vi "Graph.vi"(8 "error in (no error)":errorcluster, 11 "Message Queues":T1) -> ()   [LabVIEW 2023, in "Weather Monitor Views.lvlib"]
doc: "Calls the Weather Monitor web service with different content-types and displays the raw data that is returned."
uses:
  Weather Monitor Views.lvlib
  support/Message Queue/All Message Queues.ctl
  support/Message Queue/Message Cluster.ctl
  Request/Response Data.ctl
  <vilib>/wsapi/NI_WebServices.lvlib
  support/Message Queue/Weather Message Queue.lvlib
  Weather Request Loop.lvlib
  support/User Event - Stop/Weather User Event - Stop.lvlib
panel:
  in  "Close button":bool
  out "Weather data":picture
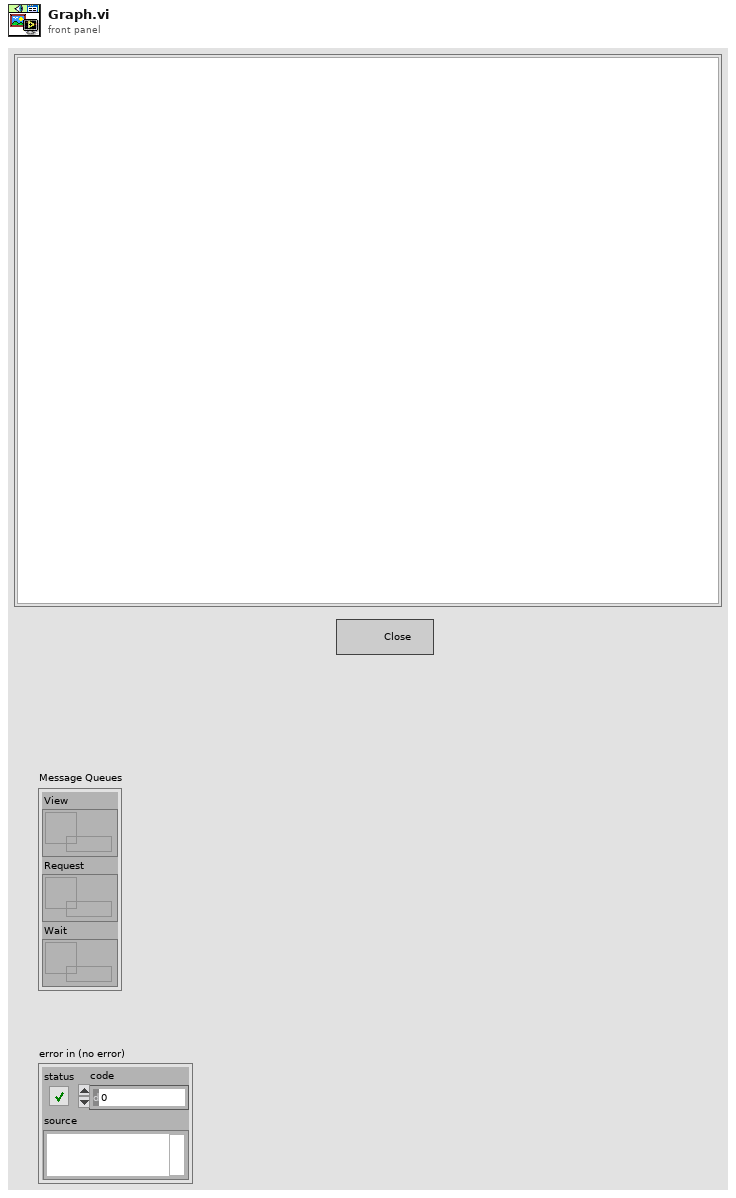
[diagram p1: front panel]
types:
  T1 = typedef "Weather Message Queue.lvlib/All Message Queues.ctl" = cluster{"View":refnum<queue>, "Request":refnum<queue>, "Wait":refnum<queue>}
  T2 = typedef "Weather Request Loop.lvlib/Response Data.ctl" = cluster{"Response Code":u16, "Body":string, "Headers":variant, "error":errorcluster}
  T3 = typedef "imagedata.ctl" = cluster{"image type":i32, "image depth":i32, "image":u8[], "mask":u8[], "colors":u32[], "Rectangle":cluster{"left":i16, "top":i16, "right":i16, "bottom":i16}}
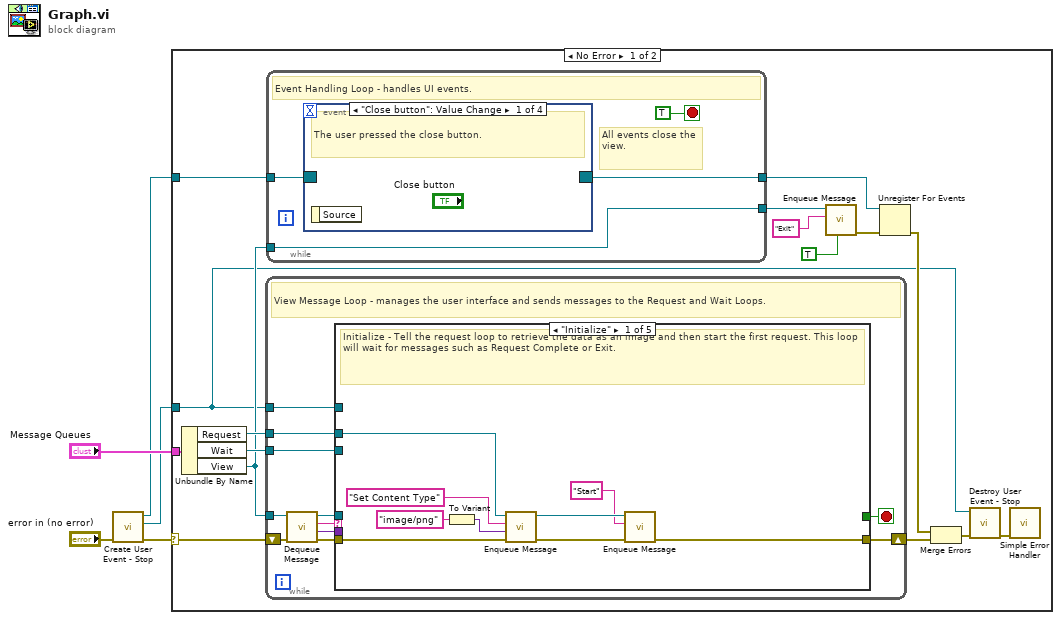
[diagram p0: block diagram]
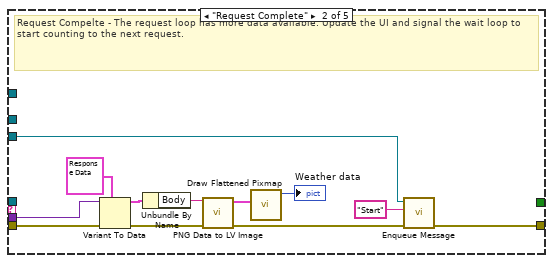
[diagram p2: hidden frame]
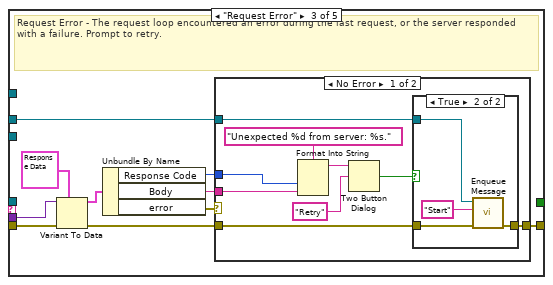
[diagram p3: hidden frame]
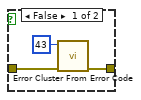
[diagram p4: hidden frame]
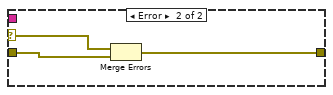
[diagram p5: hidden frame]
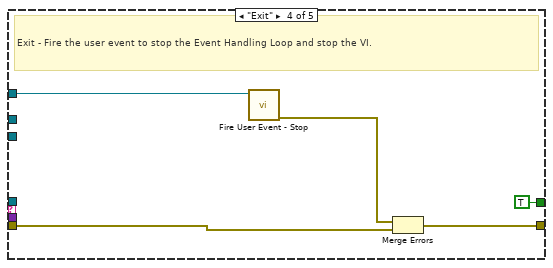
[diagram p6: hidden frame]
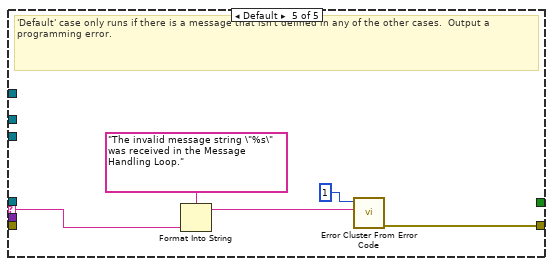
[diagram p7: hidden frame]
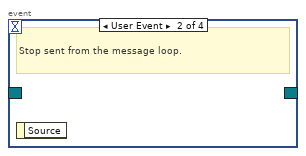
[diagram p8: hidden frame]
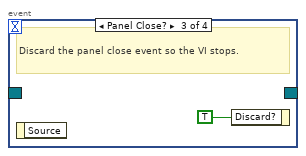
[diagram p9: hidden frame]
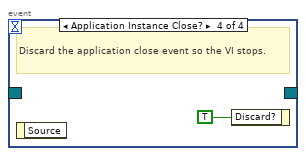
[diagram p10: hidden frame]
diagram:
  n1 = call "Create User Event - Stop.vi"("error in (no error)"="error in (no error)") -> ("error out"=w3:errorcluster, "User Event - Stop"=w1:refnum<user-event>, "Stop Event Registration Refnum"=w2:refnum<event-registration>)  [unwired: 8 in]
  n2 = case shown="No Error" w3 {
    selector: w3 -> [w16 _]
    tunnel: "Message Queues" -> [w21 _]
    tunnel: w2 -> [w15 _]
    tunnel: w1 -> [w10 _]
    frame No Error {
      n3 = Unbundle By Name(w21) -> ("Request"=w20:refnum<queue>, "Wait"=w19:refnum<queue>, "View"=w18:refnum<queue>)
      n4 = while {
        tunnel: w20 -> [w24]
        tunnel: w19 -> [w25]
        tunnel: w18 -> [w32]
        shift-right: [w26] -> w17
        shift-left: w16 -> [w31]
        tunnel: w10 -> [w22]
        stop <- w23 stop-if-true
        # "View Message Loop - manages the user interface and sends messages to the Request and Wait Loops."
        n5 = call "Dequeue Message.vi"("error in (no error)"=w31, "Message Queue"=w32) -> ("error out"=w27:errorcluster, "Message Data"=w28:variant, "Message"=w30:string, "dup Message Queue"=w29:refnum<queue>)  [unwired: 6 in]
        n6 = case shown="\"Initialize\"" w30 {
          selector: w30 -> [_ _ _ _ w89]
          tunnel: w29 -> [_ _ _ _ _]
          tunnel: w28 -> [_ w52 w62 _ _]
          tunnel: w27 -> [w41 w53 w63 w83 _]
          tunnel: [w33 w44 w55 w84 w88] -> w26
          tunnel: w25 -> [_ w43 _ _ _]
          tunnel: w24 -> [w40 _ w54 _ _]
          tunnel: [_ _ _ TRUE _] -> w23
          tunnel: w22 -> [_ _ _ w86 _]
          frame "Initialize" {
            # "Initialize - Tell the request loop to retrieve the data as an image and then start the first request. This loop will wait for messages such as Request Complete or Exit."
            n7 = To Variant(anything="image/png") -> (Variant=w37:variant)
            n8 = call "Enqueue Message.vi"("error in (no error)"=w41, "Message Data"=w37, "Message"="Set Content Type", "Message Queue"=w40) -> ("error out"=w35:errorcluster, "dup Message Queue"=w36:refnum<queue>)  [unwired: 6 in]
            n9 = call "Enqueue Message.vi"("error in (no error)"=w35, "Message"="Start", "Message Queue"=w36) -> ("error out"=w33:errorcluster)  [unwired: 7 in, 1 out]
          }
          frame "Request Complete" {
            # "Request Compelte - The request loop has more data available. Update the UI and signal the wait loop to start counting to the next request."
            n10 = Variant To Data(error in=w53, type=T2 {"Response Code"=0, "Body"="", "Headers"=variant, "error"={"status"=FALSE, "code"=0, "source"=""}} ("Response Data"), Variant=w52) -> (data=w48:T2, error out=w46:errorcluster)
            n11 = Unbundle By Name(w48) -> ("Body"=w47:string)
            n12 = call <vilib>:"PNG Data to LV Image.vi"("error in (no error)"=w46, "png data"=w47) -> ("error out"=w45:errorcluster, "image data"=w50:T3)  [unwired: 8 in]
            n13 = call <vilib>:"Draw Flattened Pixmap.vi"("image data"=w50) -> ("new picture"=→"Weather data":picture)  [unwired: 8 in]
            n14 = call "Enqueue Message.vi"("error in (no error)"=w45, "Message"="Start", "Message Queue"=w43) -> ("error out"=w44:errorcluster)  [unwired: 7 in, 1 out]
          }
          frame "Request Error" {
            # "Request Error - The request loop encountered an error during the last request, or the server responded with a failure. Prompt to retry."
            n15 = Variant To Data(error in=w63, type=T2 {"Response Code"=0, "Body"="", "Headers"=variant, "error"={"status"=FALSE, "code"=0, "source"=""}} ("Response Data"), Variant=w62) -> (data=w60:T2, error out=w57:errorcluster)
            n16 = Unbundle By Name(w60) -> ("Response Code"=w59:u16, "Body"=w58:string, "error"=w56:errorcluster)
            n17 = case shown="No Error" w56 {
              selector: w56 -> [_ w82]
              tunnel: w59 -> [w69 _]
              tunnel: w58 -> [w68 _]
              tunnel: w57 -> [w67 w80]
              tunnel: [w66 w81] -> w55
              tunnel: w54 -> [w65 _]
              frame No Error {
                n18 = Format Into String(format string="Unexpected %d from server: %s.", w69, w68) -> (resulting string=w71:string)  [unwired: 2 in, 1 out]
                n19 = Two Button Dialog(message=w71, 2:"Retry" ("T button name (\"OK\")")) -> (T button?=w64:bool)  [unwired: 1 in]
                n20 = case shown="True" w64 {
                  tunnel: w67 -> [w74 w79]
                  tunnel: [w75 w78] -> w66
                  tunnel: w65 -> [_ w77]
                  frame False {
                    n21 = call <vilib>:"Error Cluster From Error Code.vi"("error in (no error)"=w74, "error code (0)"=43) -> ("error out"=w75:errorcluster)  [unwired: 7 in]
                  }
                  frame True {
                    n22 = call "Enqueue Message.vi"("error in (no error)"=w79, "Message"="Start", "Message Queue"=w77) -> ("error out"=w78:errorcluster)  [unwired: 7 in, 1 out]
                  }
                }
              }
              frame Error {
                n23 = Merge Errors(w82, w80) -> (w81:errorcluster)
              }
            }
          }
          frame "Exit" {
            # "Exit - Fire the user event to stop the Event Handling Loop and stop the VI."
            n24 = call "Fire User Event - Stop.vi"("User Event - Stop"=w86) -> ("error out"=w85:errorcluster)  [unwired: 10 in]
            n25 = Merge Errors(w85, w83) -> (w84:errorcluster)
          }
          frame Default {
            # "'Default' case only runs if there is a message that isn't defined in any of the other cases.  Output a programming error."
            n26 = Format Into String(format string="The invalid message string \"%s\" was received in the Message Handling Loop." ("Unknown Message Error Text"), w89) -> (resulting string=w90:string)  [unwired: 2 in, 1 out]
            n27 = call <vilib>:"Error Cluster From Error Code.vi"("error message (\"\")"=w90, "error code (0)"=1) -> ("error out"=w88:errorcluster)  [unwired: 7 in]
          }
        }
      }
      n28 = while {
        tunnel: w18 -> [w93]
        tunnel: w15 -> [w95]
        tunnel: [w94] -> w13
        tunnel: [w93] -> w6
        stop <- TRUE stop-if-true
        # "All events close the view."
        # "Event Handling Loop - handles UI events."
        n29 = event shown="[0] \"Close button\": Value Change" {
          selector: w95 -> [_ _ _ _]
          dyn-events: [_ _ _ _] -> w94
          timeout: _ -> [_ _ _ _]
          event "Close button": Value Change {
            # "The user pressed the close button."
            n30 = event-data() -> ()  [unwired: 1 in, 1 out]
          }
          event User Event {
            # "Stop sent from the message loop."
            n31 = event-data() -> ()  [unwired: 1 in, 1 out]
          }
          event Panel Close? {
            # "Discard the panel close event so the VI stops."
            n32 = event-data() -> ()  [unwired: 1 in, 1 out]
            n33 = event-data("Discard?"=TRUE) -> ()  [unwired: 1 in, 1 out]
          }
          event Application Instance Close? {
            # "Discard the application close event so the VI stops."
            n34 = event-data() -> ()  [unwired: 1 in, 1 out]
            n35 = event-data("Discard?"=TRUE) -> ()  [unwired: 1 in, 1 out]
          }
        }
      }
      n36 = call "Enqueue Message.vi"("Priority Message? (F)"=TRUE, "Message"="Exit", "Message Queue"=w6) -> ("error out"=w7:errorcluster)  [unwired: 7 in, 1 out]
      n37 = Unregister For Events(event registration refnum=w13, error in=w7) -> (error out=w14:errorcluster)
      n38 = Merge Errors(w14, w17) -> (w12:errorcluster)
      n39 = call "Destroy User Event - Stop.vi"("error in (no error)"=w12, "User Event - Stop"=w10) -> ("error out"=w11:errorcluster)  [unwired: 9 in]
      n40 = call <vilib>:"Simple Error Handler.vi"("error in (no error)"=w11) -> ()  [unwired: 4 in, 5 out]
    }
    frame Error {
    }
  }
